vi "Hz (SubVI).vi"() -> (0 "Hz":dbl)   [LabVIEW 2015]
panel:
  out "x/y":dbl
  in  "정지":bool
  out "Elapsed Time (s)":dbl caption="경과 시간(초)"
  in  "현재 시간":u32
  in  "이전 시간":u32
  out "Hz1":dbl
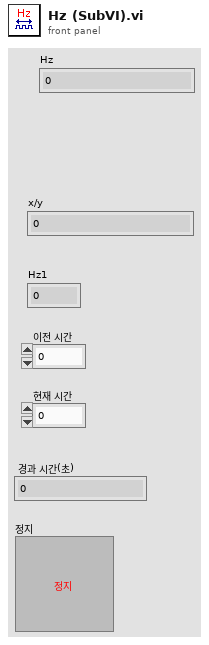
[diagram p1: front panel]
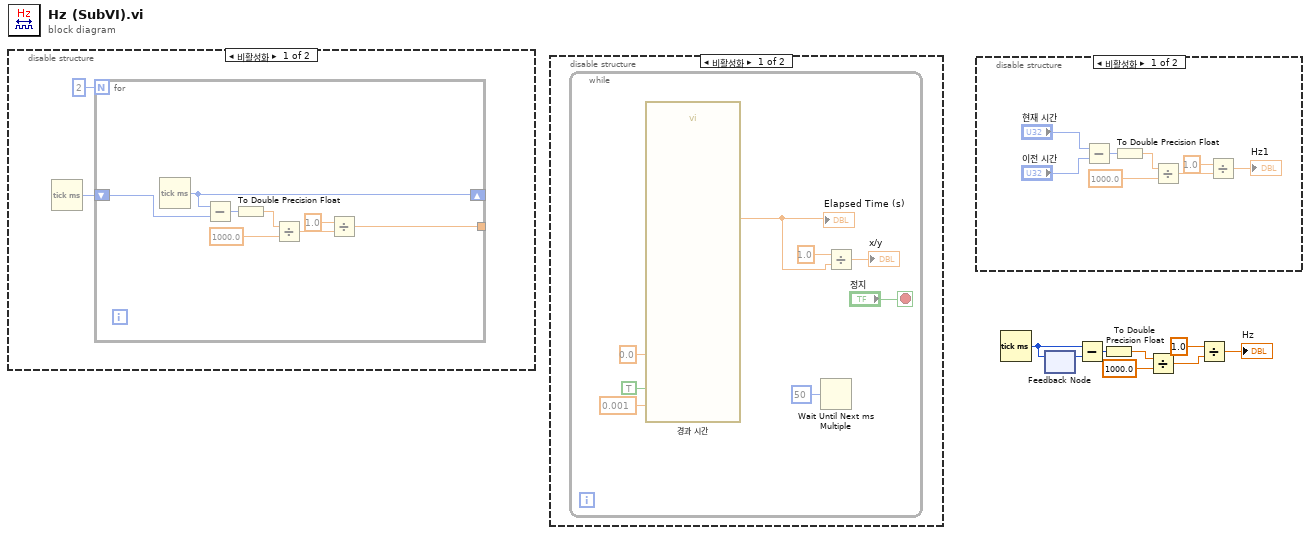
[diagram p0: block diagram]
diagram:
  n1 = disable-structure shown="비활성화" {
    frame Disabled {
      n2 = Tick Count (ms)() -> (millisecond timer value=w10:u32)
      n3 = for {
        N: 2 -> [_]
        shift-right: [w18] -> _
        shift-left: w10 -> [w17]
        tunnel: [w11] -> _
        n4 = Tick Count (ms)() -> (millisecond timer value=w18:u32)
        n5 = Subtract(x=w18, y=w17) -> (x-y=w12:u32)
        n6 = To Double Precision Float(number=w12) -> (double precision float=w13:dbl)
        n7 = Divide(x=w13, y=1000.0) -> (x/y=w14:dbl)
        n8 = Divide(x=1.0, y=w14) -> (x/y=w11:dbl)
      }
    }
    frame Enabled {
    }
  }
  n9 = disable-structure shown="비활성화" {
    frame Disabled {
      n10 = while {
        stop <- "정지" stop-if-true
        n11 = call "경과 시간"("Time Target (s)"=0.001, "Auto Reset"=TRUE, "Set Start Time (s)"=0.0) -> ("Elapsed Time (s)"=w20:dbl)  [unwired: 9 in, 7 out]
        "Elapsed Time (s)" <- w20
        n12 = Wait Until Next ms Multiple(millisecond multiple=u32 50 ("ms 배수")) -> ()  [unwired: 1 out]
        n13 = Divide(x=1.0, y=w20) -> (x/y=→"x/y":dbl)
      }
    }
    frame Enabled {
    }
  }
  n14 = disable-structure shown="비활성화" {
    frame Disabled {
      n15 = Subtract(x="현재 시간", y="이전 시간") -> (x-y=w30:u32)
      n16 = To Double Precision Float(number=w30) -> (double precision float=w31:dbl)
      n17 = Divide(x=w31, y=1000.0) -> (x/y=w32:dbl)
      n18 = Divide(x=1.0, y=w32) -> (x/y=→"Hz1":dbl)
    }
    frame Enabled {
    }
  }
  n19 = Tick Count (ms)() -> (millisecond timer value=w8:u32)
  n20 = feedback #1() -> (w7:u32)  [unwired: 1 in]
  n21 = feedback-in #1(w8) -> ()
  n22 = Subtract(x=w8, y=w7) -> (x-y=w6:u32)
  n23 = To Double Precision Float(number=w6) -> (double precision float=w4:dbl)
  n24 = Divide(x=w4, y=1000.0) -> (x/y=w3:dbl)
  n25 = Divide(x=1.0, y=w3) -> (x/y=→"Hz":dbl)
